vi "Stop Module.vi"(7 "Connection Name":string, 8 "error in (no error)":errorcluster, 9 "Wait for Module to stop? (F)":bool, 10 "Origin":string, 11 "Module ID":i32=-1) -> (0 "error out":errorcluster)   [LabVIEW 2017, in "SSH.lvlib"]
doc: "Send the Stop request to the Module's Main.vi.\n_____\nBased on Delacor QMH Project Template 4.2.1.64."
uses:
  SSH.lvlib
  Stop Argument--cluster.ctl
  <vilib>/event_ctls.llb/usereventprio.ctl
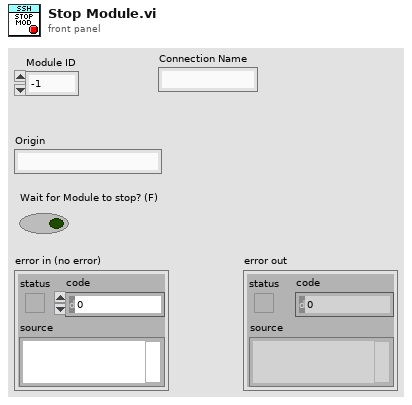
[diagram p1: front panel]
types:
  T1 = typedef "SSH.lvlib/Stop Argument--cluster.ctl" = cluster{"Module ID":i32, "Origin":string, "Exit via Stop Module Req?":bool, "Wait for Module to stop?":bool}
  T2 = typedef "SSH.lvlib/Request Events--cluster.ctl" = cluster{"Stop Module":refnum<user-event>, "Show Panel":refnum<user-event>, "Hide Panel":refnum<user-event>, "Show Diagram":refnum<user-event>, "Get Module Execution Status":refnum<user-event>, "Write Command":refnum<user-event>}
  T3 = typedef "usereventprio.ctl" = enum32{"high priority", "normal priority"}
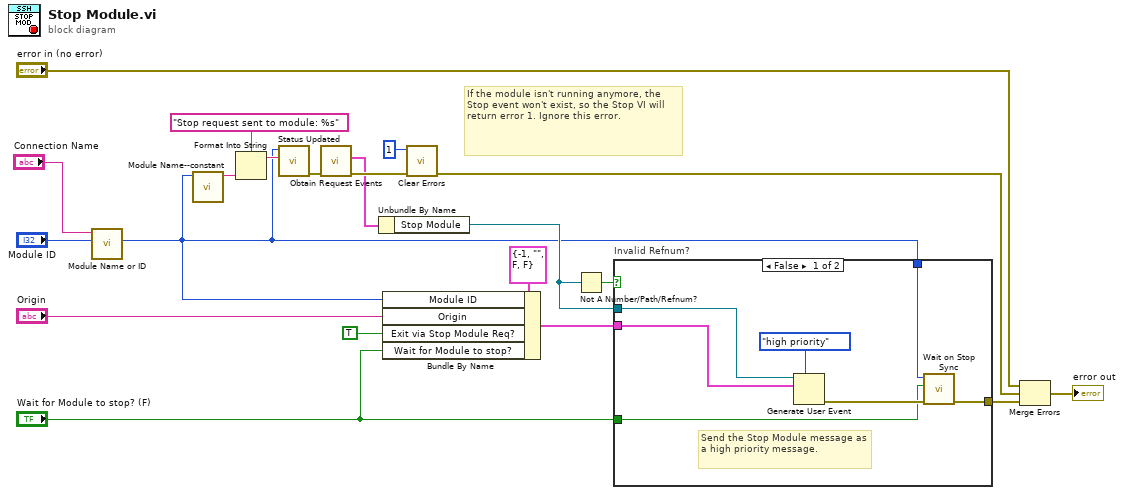
[diagram p0: block diagram]
diagram:
  # "If the module isn't running anymore, the Stop event won't exist, so the Stop VI will return error 1. Ignore this error."
  n1 = call "Module Name or ID.vi"("Module ID in"="Module ID", "Connection Name"="Connection Name") -> ("Module ID out"=w2:i32)  [unwired: 9 in]
  n2 = call "Module Name--constant.vi"("Module ID"=w2) -> ("Module Name"=w18:string)  [unwired: 10 in]
  n3 = Format Into String(format string="Stop request sent to module: %s", w18) -> (resulting string=w19:string)  [unwired: 2 in, 1 out]
  n4 = call "Status Updated.vi"("Status"=w19, "Module ID"=w2) -> ("error out"=w11:errorcluster)  [unwired: 9 in]
  n5 = call "Obtain Request Events.vi"("error in (no error)"=w11) -> ("error out"=w10:errorcluster, "SSH Request Events"=w8:T2)  [unwired: 9 in]
  n6 = Unbundle By Name(w8) -> ("Stop Module"=w13:refnum<user-event>)
  n7 = Bundle By Name(cluster=T1 {"Module ID"=-1, "Origin"="", "Exit via Stop Module Req?"=FALSE, "Wait for Module to stop?"=FALSE} ("event data"), "Module ID"=w2, "Origin"="Origin", "Exit via Stop Module Req?"=TRUE, "Wait for Module to stop?"="Wait for Module to stop? (F)") -> (w12:T1)
  n8 = call <vilib>:"Clear Errors.vi"("error in (no error)"=w10, "specific error code to clear (0: all)"=1) -> ("error out"=w7:errorcluster)  [unwired: 4 in, 1 out]
  n9 = Not A Number/Path/Refnum?(number/path/refnum=w13) -> (NaN/Path/Refnum?=w14:bool)
  n10 = case "Invalid Refnum?" shown="False" w14 {
    tunnel: [w24 _] -> w6
    tunnel: w12 -> [w28 _]
    tunnel: w13 -> [w27 _]
    tunnel: w2 -> [w23 _]
    tunnel: "Wait for Module to stop? (F)" -> [w22 _]
    frame False {
      # "Send the Stop Module message as a high priority message."
      n11 = Generate User Event(priority (normal)=usereventprio."high priority", user event=w27, event data cluster=w28) -> (error out=w25:errorcluster)  [unwired: 1 in, 1 out]
      n12 = call "Wait on Stop Sync.vi"("error in (no error)"=w25, "Wait for Module to stop?"=w22, "Module ID"=w23) -> ("error out"=w24:errorcluster)  [unwired: 8 in]
    }
    frame True {
      # "Module is exiting. No need to send the standard \"not running\" error that is sent in other request VIs."
    }
  }
  n13 = Merge Errors("error in (no error)", w7, w6) -> (→"error out":errorcluster)
